vi "K2000.vi"(8 "error constant":errorcluster) -> (0 "error constant 2":errorcluster)   [LabVIEW 2019]
uses:
  <vilib>/myRIO/Instrument Drivers/Onboard IO/DIO/typedefs/DIO Reference.ctl
  <vilib>/myRIO/Common/Instrument Driver Framework/Utilities/typedefs/myRIO Generic Hardware Reference.ctl
  <vilib>/myRIO/Common/Instrument Driver Framework/Utilities/typedefs/Hardware Version Enum.ctl
  <vilib>/myRIO/Common/Instrument Driver Framework/Utilities/typedefs/myRIO v1.0 Reference.ctl
  <vilib>/myRIO/Common/Instrument Driver Framework/Utilities/typedefs/Generic FPGA Reference.ctl
  <vilib>/myRIO/Common/Instrument Driver Framework/myRIO v1.0/DIO/typedefs/DIO Channels List.ctl
  <vilib>/myRIO/Common/Instrument Driver Framework/myRIO v1.0/DIO/typedefs/DIO Channels Enum.ctl
  <vilib>/userDefined/High Color/nirio_resource_hc.ctl
  <vilib>/myRIO/Common/Instrument Driver Framework/Utilities/vis/Is FPGA Ref Available.vi
  <vilib>/myRIO/Common/Instrument Driver Framework/myRIO v1.0/DIO/vis/myRIO v1.1 Open DIO.vi
  <vilib>/myRIO/Instrument Drivers/Onboard IO/DIO/vis/Write.vi
  <vilib>/myRIO/Common/Instrument Driver Framework/Utilities/vis/Validate Channels.vi
  <vilib>/myRIO/Common/Instrument Driver Framework/myRIO v1.0/DIO/vis/myRIO v1.0 Reserve DIO.vi
  <vilib>/myRIO/Common/Instrument Driver Framework/myRIO v1.0/Resource Manager/vis/myRIO v1.0 Reserve Channel List.vi
  <vilib>/myRIO/Common/Instrument Driver Framework/myRIO v1.0/DIO/vis/myRIO v1.0 Build MUX Configuration DIO.vi
  <vilib>/myRIO/Common/Instrument Driver Framework/myRIO v1.0/Resource Manager/vis/myRIO v1.0 Reserve Channel.vi
  <vilib>/myRIO/Common/Instrument Driver Framework/myRIO v1.0/Resource Manager/vis/myRIO v1.0 Unreserve Channel.vi
  <vilib>/myRIO/Common/Instrument Driver Framework/myRIO v1.0/Resource Manager/vis/myRIO v1.0 Create Configuration List.vi
  <vilib>/myRIO/Common/Instrument Driver Framework/myRIO v1.0/Resource Manager/vis/myRIO v1.0 Build Mutex Name.vi
  <vilib>/Utility/VariantDataType/GetNumericInfo.vi
  <vilib>/Utility/error.llb/Error Cluster From Error Code.vi
  <vilib>/myRIO/Common/Instrument Driver Framework/myRIO v1.0/myRIO v1.1 Open.vi
  <vilib>/myRIO/Common/Instrument Driver Framework/Utilities/vis/IO Manager.vi
  <vilib>/myRIO/Common/Instrument Driver Framework/Utilities/vis/Configuration Manager.vi
  <vilib>/myRIO/Common/Instrument Driver Framework/myRIO v1.0/Resource Manager/vis/myRIO v1.0 Configure IO.vi
  <vilib>/myRIO/Common/Instrument Driver Framework/myRIO v1.0/myRIO v1.0 Close.vi
  <vilib>/myRIO/Common/Instrument Driver Framework/myRIO v1.0/DIO/vis/myRIO v1.0 Write DIO.vi
  <vilib>/myRIO/Express VI/Onboard Devices/LED/LED Express VI.xnode
  <vilib>/myRIO/Instrument Drivers/Onboard IO/DIO/vis/myRIO DIO Open.xnode
  <vilib>/myRIO/Instrument Drivers/Onboard IO/DIO/DIO.lvlib
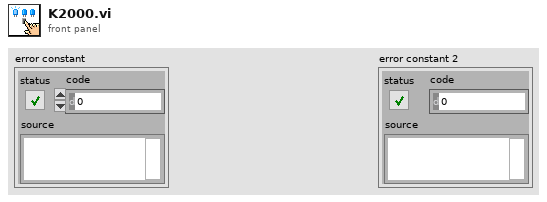
[diagram p1: front panel]
types:
  T1 = typedef "DIO.lvlib/DIO Reference.ctl" = cluster{"myRIO Reference":T2, "DIO Channels List":T6}
  T2 = typedef "myRIO Generic Hardware Reference.ctl" = cluster{"myRIO Model":T3, "myRIO Hardware Reference":T4}
  T3 = typedef "Hardware Version Enum.ctl" = enum16{"Unknown", "myRIO-1900", "myRIO-1950", "roboRIO", "NI ELVIS RIO CM", "ELVIS III"}
  T4 = typedef "myRIO v1.0 Reference.ctl" = cluster{"Generic FPGA Reference":T5, "Allow multiple opens":bool}
  T5 = typedef "Generic FPGA Reference.ctl" = refnum<k20>
  T6 = typedef "DIO Channels List.ctl" = T7[]
  T7 = typedef "DIO Channels Enum.ctl" = enum16{"Not Connected", "C/DIO0", "C/DIO1", "C/DIO2", "C/DIO3", "C/DIO4", "C/DIO5", "C/DIO6", "C/DIO7", "A/DIO0", "A/DIO1", "A/DIO2", "A/DIO3", "A/DIO4", "A/DIO5", "A/DIO6", "A/DIO7", "A/DIO8", "A/DIO9", "A/DIO10", "A/DIO11", "A/DIO12", "A/DIO13", "A/DIO14", "A/DIO15", "A/DIO16", "A/DIO17", "A/DIO18", "A/DIO19", "B/DIO0", "B/DIO1", "B/DIO2", "B/DIO3", "B/DIO4", "B/DIO5", "B/DIO6", "B/DIO7", "B/DIO8", "B/DIO9", "B/DIO10", "B/DIO11", "B/DIO12", "B/DIO13", "B/DIO14", "B/DIO15", "B/DIO16", "B/DIO17", "B/DIO18", "B/DIO19", "LED0", "LED1", "LED2", "LED3", "Button0", "DIO/DIO0", "DIO/DIO1", "DIO/DIO2", "DIO/DIO3", "DIO/DIO4", "DIO/DIO5", "DIO/DIO6", "DIO/DIO7", "DIO/DIO8", "DIO/DIO9", "SPI/CS0", "SPI/CS1", "SPI/CS2", "SPI/CS3", "LED RADIO (Green)", "LED RADIO (Red)", "LED COMM (Green)", "LED COMM (Red)", "LED MODE (Green)", "LED MODE (Red)"}
  T8 = typedef "nirio_resource_hc.ctl" = tag
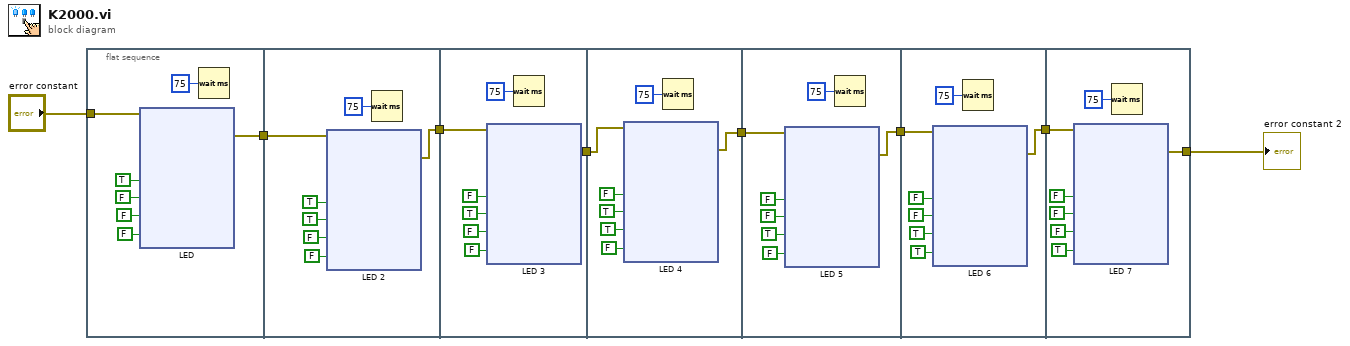
[diagram p0: block diagram]
diagram:
  n1 = flat-sequence {
    tunnel: [w11] -> w8
    tunnel: "error constant" -> [w10]
    tunnel: w8 -> [w56]
    tunnel: [w55] -> w7
    tunnel: w7 -> [w101]
    tunnel: [w100] -> w6
    tunnel: w6 -> [w146]
    tunnel: [w145] -> w5
    tunnel: w5 -> [w191]
    tunnel: [w190] -> w4
    tunnel: w4 -> [w236]
    tunnel: [w235] -> w3
    tunnel: w3 -> [w281]
    tunnel: [w280] -> w1
    frame #0 {
      n2 = xnode "LED"("L0"=TRUE, "L1"=FALSE ("L0"), "L2"=FALSE ("L0"), "L3"=FALSE ("L0"), "error in (no error)"=w10) -> ("error out"=w11:errorcluster)
      n3 = Wait (ms)(milliseconds to wait=u32 75) -> ()  [unwired: 1 out]
    }
    frame #1 {
      n4 = xnode "LED 2"("L0"=TRUE, "L1"=TRUE ("L0"), "L2"=FALSE ("L0"), "L3"=FALSE ("L0"), "error in (no error)"=w56) -> ("error out"=w55:errorcluster)
      n5 = Wait (ms)(milliseconds to wait=u32 75) -> ()  [unwired: 1 out]
    }
    frame #2 {
      n6 = xnode "LED 3"("L0"=FALSE, "L1"=TRUE ("L0"), "L2"=FALSE ("L0"), "L3"=FALSE ("L0"), "error in (no error)"=w101) -> ("error out"=w100:errorcluster)
      n7 = Wait (ms)(milliseconds to wait=u32 75) -> ()  [unwired: 1 out]
    }
    frame #3 {
      n8 = xnode "LED 4"("L0"=FALSE, "L1"=TRUE ("L0"), "L2"=TRUE ("L0"), "L3"=FALSE ("L0"), "error in (no error)"=w146) -> ("error out"=w145:errorcluster)
      n9 = Wait (ms)(milliseconds to wait=u32 75) -> ()  [unwired: 1 out]
    }
    frame #4 {
      n10 = xnode "LED 5"("L0"=FALSE, "L1"=FALSE ("L0"), "L2"=TRUE ("L0"), "L3"=FALSE ("L0"), "error in (no error)"=w191) -> ("error out"=w190:errorcluster)
      n11 = Wait (ms)(milliseconds to wait=u32 75) -> ()  [unwired: 1 out]
    }
    frame #5 {
      n12 = xnode "LED 6"("L0"=FALSE, "L1"=FALSE ("L0"), "L2"=TRUE ("L0"), "L3"=TRUE ("L0"), "error in (no error)"=w236) -> ("error out"=w235:errorcluster)
      n13 = Wait (ms)(milliseconds to wait=u32 75) -> ()  [unwired: 1 out]
    }
    frame #6 {
      n14 = xnode "LED 7"("L0"=FALSE, "L1"=FALSE ("L0"), "L2"=FALSE ("L0"), "L3"=TRUE ("L0"), "error in (no error)"=w281) -> ("error out"=w280:errorcluster)
      n15 = Wait (ms)(milliseconds to wait=u32 75) -> ()  [unwired: 1 out]
    }
  }
  "error constant 2" <- w1
